vi "TrapXYZStiffness.vi"(9 "XYZ Squared":cluster{i16, i16, i16}[](array[cluster]), 11 "XYZ":cluster{i16, i16, i16}[](array[cluster])) -> (2 "XYZ St. dev.":cluster{dbl, dbl, dbl})   [LabVIEW 2018]
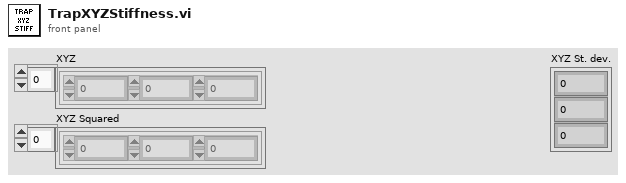
[diagram p1: front panel]
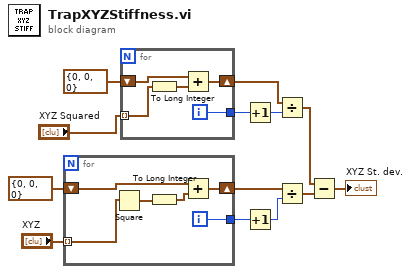
[diagram p0: block diagram]
diagram:
  n1 = for {
    tunnel: "XYZ" -> [w18] mode=indexing
    shift-right: [w16] -> w10
    shift-left: cluster{i32, i32, i32} {0, 0, 0} -> [w19]
    tunnel: [w15] -> w11
    i -> [w15]
    n2 = Square(x=w18) -> (x^2=w14:cluster{i16, i16, i16})
    n3 = To Long Integer(number=w14) -> (32bit integer=w17:cluster{i32, i32, i32})
    n4 = Add(x=w19, y=w17) -> (x+y=w16:cluster{i32, i32, i32})
  }
  n5 = for {
    tunnel: "XYZ Squared" -> [w23] mode=indexing
    shift-right: [w21] -> w5
    shift-left: cluster{i32, i32, i32} {0, 0, 0} -> [w24]
    tunnel: [w20] -> w4
    i -> [w20]
    n6 = To Long Integer(number=w23) -> (32bit integer=w22:cluster{i32, i32, i32})
    n7 = Add(x=w24, y=w22) -> (x+y=w21:cluster{i32, i32, i32})
  }
  n8 = Increment(x=w4) -> (x+1=w6:i32)
  n9 = Increment(x=w11) -> (x+1=w9:i32)
  n10 = Divide(x=w5, y=w6) -> (x/y=w3:cluster{dbl, dbl, dbl})
  n11 = Divide(x=w10, y=w9) -> (x/y=w2:cluster{dbl, dbl, dbl})
  n12 = Subtract(x=w3, y=w2) -> (x-y=→"XYZ St. dev.":cluster{dbl, dbl, dbl})
